vi "flight_time_05_12_v2.vi"() -> ()   [LabVIEW 2013]
uses:
  <vilib>/Instr/_visa.llb/VISA Configure Serial Port (Instr).vi
  <vilib>/Analysis/NI_AALBase.lvlib
panel:
  in  "lock":u8=3
  out "avg_cell4":dbl
  out "avg_cell3":dbl
  out "avg_cell2":dbl
  out "avg_cell1":dbl
  in  "stop":bool
  in  "Pcell1":u32[](array[numeric])
  in  "Pcell2":u32[](array[numeric])
  in  "Pcell3":u32[](array[numeric])
  in  "Pcell4":u32[](array[numeric])
  out "time":u32[](graph)
  in  "Tab Control":enum32{"Calibração", "filter"}(tab)
  out "raw_cell1":dbl(graph) caption="Celula 1"
  out "raw_cell2":dbl(graph) caption="Celula 2"
  out "raw_cell3":dbl(graph) caption="Celula 3"
  out "raw_cell4":dbl(graph) caption="Celula 4"
  out "state":bool
  out "calibrado1":dbl(graph) caption="Celula 1"
  out "calibrado3":dbl(graph) caption="Celula 3"
  out "calibrado2":dbl(graph) caption="Celula 2"
  out "calibrado4":dbl(graph) caption="Celula 4"
  in  "?":bool
  out "tempo de voo (ms)":dbl
  out "stop 2":dbl
  out "start":dbl
  in  "?":bool
  out "h":dbl caption="Altura (cm)"
  out "calibrado4 2":dbl(graph)
  out "flight_time_graph":dbl(graph) caption="Tempo de voo"
  out "cell":u8[](array[numeric])
  out "output_int16":i32[](array[numeric])
  out "data":u8[](array[numeric])
  in  "serial_port":refnum<visa-resource-name>="COM7" caption="Porta Serial"
  # "Aguarde 10 segundos para a calibração do sistema"
  # "Sistema calibrado e pronto para operação"
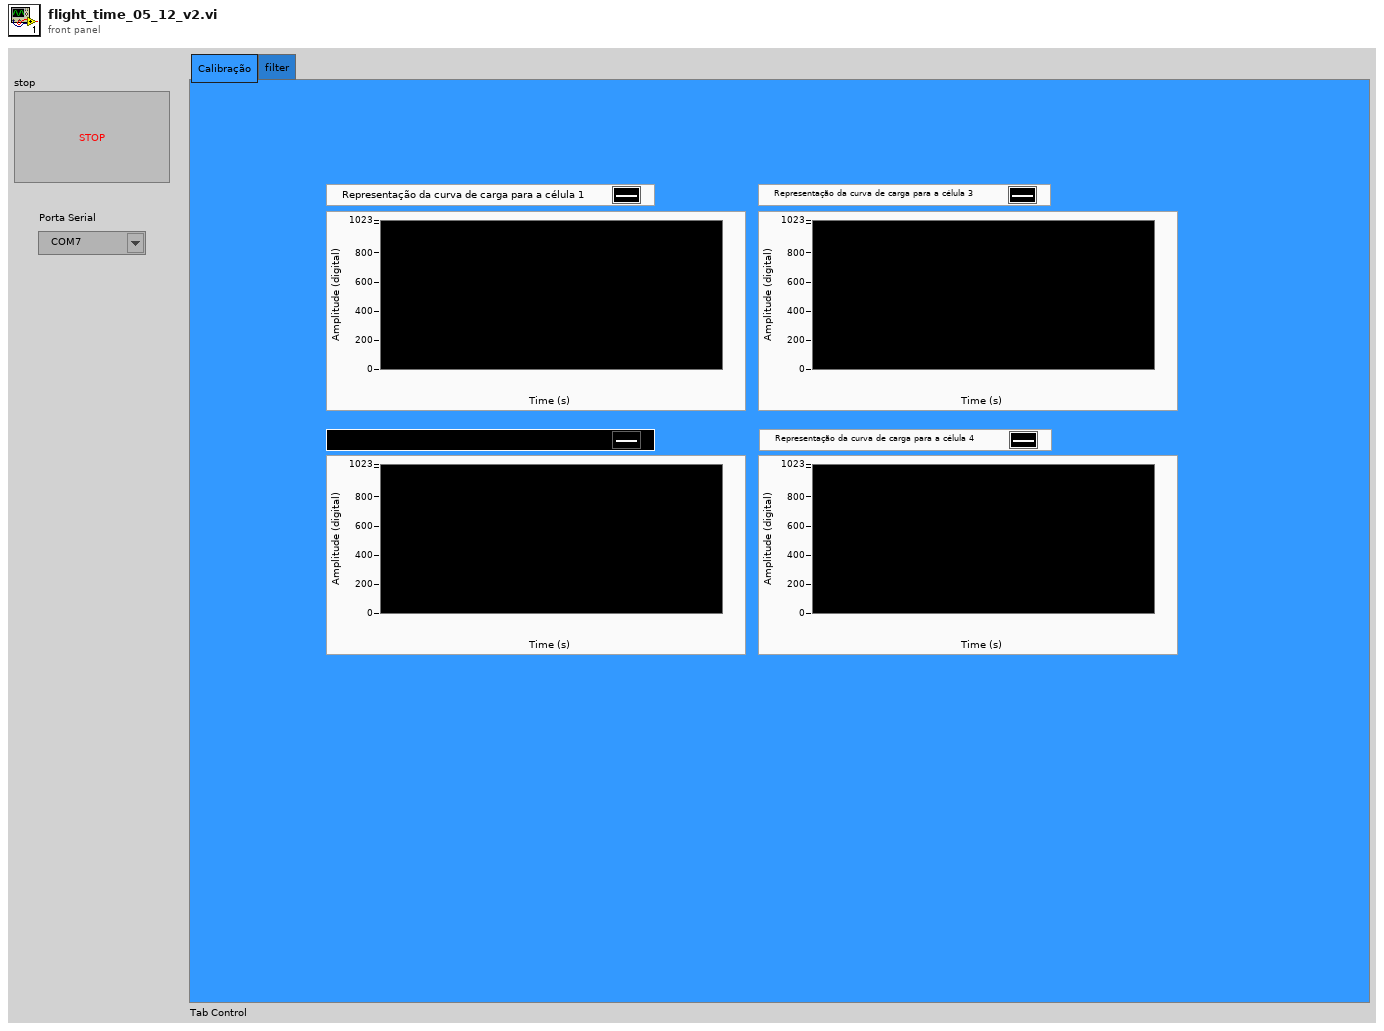
[diagram p1: front panel]
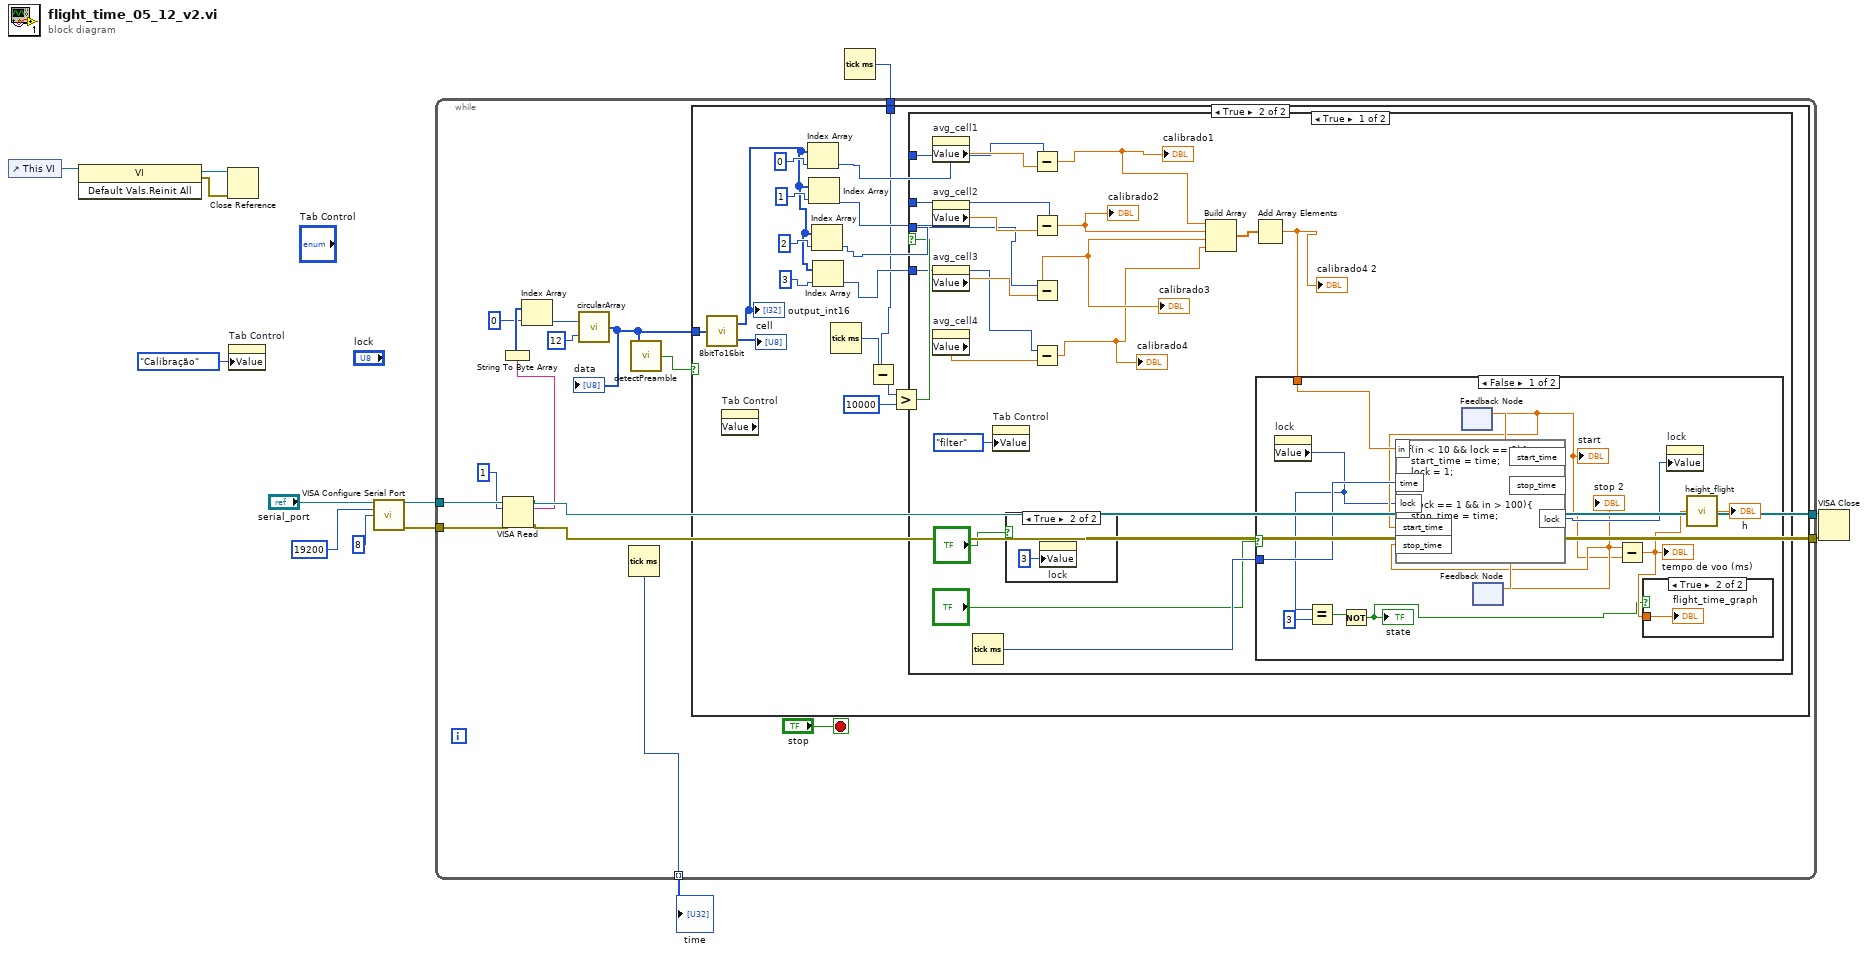
[diagram p0: block diagram]
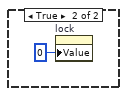
[diagram p5: hidden frame]
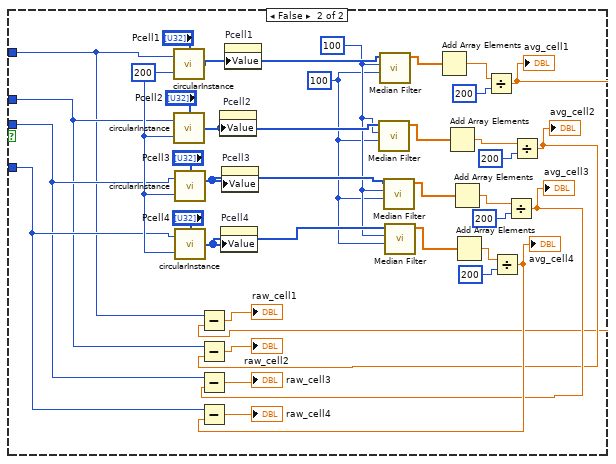
[diagram p6: hidden frame]
diagram:
  n1 = control-ref of="This VI"() -> (w3:refnum<vi>)
  n2 = invoke class="VI" method="Default Vals.Reinit All"(reference=w3) -> (reference out=w2:refnum<vi>, error out=w1:errorcluster)  [unwired: 2 in, 1 out]
  n3 = Close Reference(reference=w2, error in (no error)=w1) -> ()  [unwired: 1 out]
  n4 = property on="Tab Control" class="TabCtl (strict)"("Value"=enum32{"Calibração", "filter"}."Calibração" ("Tab Control")) -> ()  [unwired: 2 in, 2 out]
  n5 = call-poly "VISA Configure Serial Port"("VISA resource name"="serial_port", "baud rate (9600)"=u32 19200, "data bits (8)"=u16 8) -> ("VISA resource name out"=w10:refnum<visa-resource-name>, "error out"=w9:errorcluster)  [unwired: 11 in]
  n6 = Tick Count (ms)() -> (millisecond timer value=w5:u32)
  n7 = while {
    tunnel: w10 -> [w28]
    tunnel: w9 -> [w27]
    tunnel: [w25] -> w7
    tunnel: [w26] -> w8
    tunnel: [w16] -> w6 mode=indexing
    tunnel: w5 -> [w14]
    stop <- "stop" stop-if-true
    n8 = VISA Read(VISA resource name=w28, byte count=1, error in (no error)=w27) -> (VISA resource name out=w26:refnum<visa-resource-name>, read buffer=w20:string, error out=w25:errorcluster)  [unwired: 1 out]
    n9 = String To Byte Array(string=w20) -> (unsigned byte array=w23:u8[])
    n10 = Index Array(array=w23, index=0) -> (element=w17:u8)
    n11 = call "circularArray.vi"("max-size"=u8 12, "element"=w17) -> ("dataout"=w18:u8[])
    "data" <- w18
    n12 = Tick Count (ms)() -> (millisecond timer value=w16:u32)
    n13 = call "detectPreamble.vi"("data-in"=w18) -> ("detected"=w15:bool)
    n14 = case shown="True" w15 {
      tunnel: w18 -> [_ w43]
      tunnel: w14 -> [_ w32]
      frame False {
      }
      frame True {
        n15 = call "8bitTo16bit.vi"("input_byte"=w43) -> ("output_int16"=w38:i32[], "cell"=→"cell":u8[])
        "output_int16" <- w38
        n16 = property on="Tab Control" class="TabCtl (strict)" props=["Value"]() -> ()  [unwired: 2 in, 3 out]
        n17 = Index Array(array=w38, index=0) -> (element=w34:i32)
        n18 = Index Array(array=w38, index=1) -> (element=w35:i32)
        n19 = Index Array(array=w38, index=2) -> (element=w36:i32)
        n20 = Index Array(array=w38, index=3) -> (element=w37:i32)
        n21 = Tick Count (ms)() -> (millisecond timer value=w33:u32)
        n22 = Subtract(x=w33, y=w32) -> (x-y=w31:u32)
        n23 = Greater?(x=w31, y=u32 10000) -> (0:w29:bool)
        n24 = case shown="True" w29 {
          tunnel: w34 -> [w55 w82]
          tunnel: w35 -> [w52 w83]
          tunnel: w36 -> [w53 w84]
          tunnel: w37 -> [w54 w90]
          frame True {
            n25 = property on="avg_cell1" class="DigNum (strict)"() -> ("Value"=w60:dbl)  [unwired: 2 in, 2 out]
            n26 = property on="avg_cell2" class="DigNum (strict)"() -> ("Value"=w59:dbl)  [unwired: 2 in, 2 out]
            n27 = property on="avg_cell3" class="DigNum (strict)"() -> ("Value"=w58:dbl)  [unwired: 2 in, 2 out]
            n28 = property on="avg_cell4" class="DigNum (strict)"() -> ("Value"=w57:dbl)  [unwired: 2 in, 2 out]
            n29 = Tick Count (ms)() -> (millisecond timer value=w62:u32)
            n30 = property on="Tab Control" class="TabCtl (strict)"("Value"=enum32{"Calibração", "filter"}."filter" ("Tab Control")) -> ()  [unwired: 2 in, 2 out]
            n31 = case shown="True" "?" {
              frame False {
              }
              frame True {
                n32 = property on="lock" class="DigNum (strict)"("Value"=u8 3 ("lock")) -> ()  [unwired: 2 in, 2 out]
              }
            }
            n33 = Subtract(x=w55, y=w60) -> (x-y=w51:dbl)
            "calibrado1" <- w51
            n34 = Subtract(x=w52, y=w59) -> (x-y=w50:dbl)
            "calibrado2" <- w50
            n35 = Subtract(x=w53, y=w58) -> (x-y=w49:dbl)
            "calibrado3" <- w49
            n36 = Subtract(x=w54, y=w57) -> (x-y=w48:dbl)
            "calibrado4" <- w48
            n37 = Build Array(w51, w50, w49, w48) -> (w56:dbl[])
            n38 = Add Array Elements(numeric array=w56) -> (sum=w45:dbl)
            "calibrado4 2" <- w45
            n39 = case shown="False" "?" {
              tunnel: w62 -> [w76 _]
              tunnel: w45 -> [w75 _]
              frame False {
                n40 = property on="lock" class="DigNum (strict)"() -> ("Value"=w68:u8)  [unwired: 2 in, 2 out]
                n41 = Equal?(x=w68, y=u8 3) -> (x = y?=w66:bool)
                n42 = Not(x=w66) -> (.not. x?=w64:bool)
                "state" <- w64
                n43 = feedback #1() -> (w70:dbl)  [unwired: 1 in]
                "start" <- w70
                n44 = feedback #2() -> (w72:dbl)  [unwired: 1 in]
                "stop 2" <- w72
                n45 = formula code="if(in < 10 && lock == 0){\n  start_time = time;\n  lock = 1;\n}\n\nif(lock == 1 && in > 100){\n  stop_time = time;\n  lock = 0;\n}"("in"=w75, "time"=w76, "lock"=w68, "start_time"=w70, "stop_time"=w72) -> ("start_time"=w71:dbl, "stop_time"=w73:dbl, "lock"=w74:u8)
                n46 = feedback-in #1(w71) -> ()
                n47 = feedback-in #2(w73) -> ()
                n48 = Subtract(x=w72, y=w70) -> (x-y=w65:dbl)
                "tempo de voo (ms)" <- w65
                n49 = case shown="True" w64 {
                  tunnel: w65 -> [_ w77]
                  frame False {
                  }
                  frame True {
                    "flight_time_graph" <- w77
                  }
                }
                n50 = property on="lock" class="DigNum (strict)"("Value"=w74) -> ()  [unwired: 2 in, 2 out]
                n51 = call "height_flight.vi"("t"=w65) -> ("h"=→"h":dbl)
              }
              frame True {
                n52 = property on="lock" class="DigNum (strict)"("Value"=u8 0 ("input variable")) -> ()  [unwired: 2 in, 2 out]
              }
            }
          }
          frame False {
            w103 = 100 ("left rank")
            w104 = 100 ("left rank")
            w111 = i16 200 ("max-size")
            n53 = call "circularInstance.vi"("data"="Pcell1", "max-size"=w111, "element"=w82) -> ("dataout"=w108:u32[])
            n54 = call "circularInstance.vi"("data"="Pcell2", "max-size"=w111, "element"=w83) -> ("dataout"=w107:u32[])
            n55 = call "circularInstance.vi"("data"="Pcell3", "max-size"=w111, "element"=w84) -> ("dataout"=w106:u32[])
            n56 = call "circularInstance.vi"("data"="Pcell4", "max-size"=w111, "element"=w90) -> ("dataout"=w105:u32[])
            n57 = property on="Pcell2" class="Arr (strict)"("Value"=w107) -> ()  [unwired: 2 in, 2 out]
            n58 = property on="Pcell4" class="Arr (strict)"("Value"=w105) -> ()  [unwired: 2 in, 2 out]
            n59 = property on="Pcell3" class="Arr (strict)"("Value"=w106) -> ()  [unwired: 2 in, 2 out]
            n60 = property on="Pcell1" class="Arr (strict)"("Value"=w108) -> ()  [unwired: 2 in, 2 out]
            n61 = call <vilib>:"Median Filter.vi"("right rank"=w103, "left rank"=w104, "X"=w107) -> ("Filtered X"=w102:dbl[])  [unwired: 7 in, 1 out]
            n62 = call <vilib>:"Median Filter.vi"("right rank"=w103, "left rank"=w104, "X"=w108) -> ("Filtered X"=w92:dbl[])  [unwired: 7 in, 1 out]
            n63 = call <vilib>:"Median Filter.vi"("right rank"=w103, "left rank"=w104, "X"=w106) -> ("Filtered X"=w101:dbl[])  [unwired: 7 in, 1 out]
            n64 = call <vilib>:"Median Filter.vi"("right rank"=w103, "left rank"=w104, "X"=w105) -> ("Filtered X"=w91:dbl[])  [unwired: 7 in, 1 out]
            n65 = Add Array Elements(numeric array=w92) -> (sum=w99:dbl)
            n66 = Add Array Elements(numeric array=w102) -> (sum=w93:dbl)
            n67 = Add Array Elements(numeric array=w101) -> (sum=w94:dbl)
            n68 = Add Array Elements(numeric array=w91) -> (sum=w95:dbl)
            n69 = Divide(x=w99, y=i16 200 ("max-size")) -> (x/y=w85:dbl)
            "avg_cell1" <- w85
            n70 = Subtract(x=w82, y=w85) -> (x-y=→"raw_cell1":dbl)
            n71 = Divide(x=w95, y=i16 200 ("max-size")) -> (x/y=w89:dbl)
            "avg_cell4" <- w89
            n72 = Subtract(x=w90, y=w89) -> (x-y=→"raw_cell4":dbl)
            n73 = Divide(x=w94, y=i16 200 ("max-size")) -> (x/y=w87:dbl)
            "avg_cell3" <- w87
            n74 = Subtract(x=w84, y=w87) -> (x-y=→"raw_cell3":dbl)
            n75 = Divide(x=w93, y=i16 200 ("max-size")) -> (x/y=w86:dbl)
            "avg_cell2" <- w86
            n76 = Subtract(x=w83, y=w86) -> (x-y=→"raw_cell2":dbl)
          }
        }
      }
    }
  }
  "time" <- w6
  n77 = VISA Close(VISA resource name=w8, error in (no error)=w7) -> ()  [unwired: 1 out]
